vi "Auto Shooter Mode.vi"(0 "Shooter Command":T1, 7 "Current Angle":dbl, 9 "Ball Loaded?":bool) -> (8 "Secure Ball?":bool, 10 "Angle In Range?":bool, 11 "RPM Ready?":bool, 12 "Vision Target Aligned?":bool, 14 "State":T5, 15 "Shooter Ready?":bool, 16 "Left Output":dbl, 17 "Right Output":dbl, 18 "Angle Motor Output":dbl, 19 "Trigger Output":dbl)   [LabVIEW 2015]
uses:
  Common Code/Shooter State.ctl
  Common Code/Shooter Command Cluster.ctl
  Common Code/Shooter Commands.ctl
  Common Code/Shoot Modes Enum.ctl
  Common Code/Shot Type.ctl
  Common Code/Change Detect Int.vi
  Common Code/Change Detect Double.vi
  Robot Global Data.vi
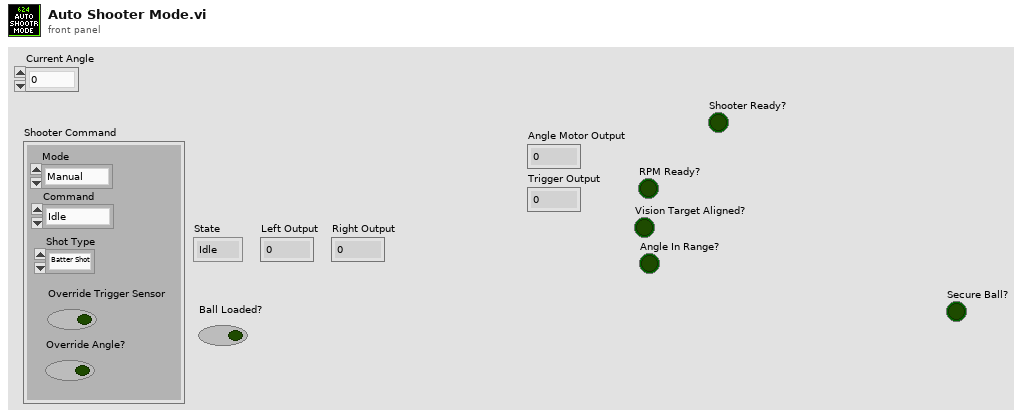
[diagram p1: front panel]
types:
  T1 = typedef "Shooter Command Cluster.ctl" = cluster{"Command":T2, "Mode":T3, "Shot Type":T4, "Override Trigger Sensor":bool, "Override Angle?":bool}
  T2 = typedef "Shooter Commands.ctl" = enum16{"Idle", "Prime Shooter", "Shoot"}
  T3 = typedef "Shoot Modes Enum.ctl" = enum16{"Manual", "Safe", "Auto"}
  T4 = typedef "Shot Type.ctl" = enum16{"Batter Shot", "Corner Shot", "Curve Shot", "Vision Shot", "Deep Middle Shot"}
  T5 = typedef "Shooter State.ctl" = enum16{"Idle", "Warmup", "Shooter Ready", "Shoot"}
  T6 = typedef "Dashboard Control Data.ctl" = cluster{"Shooter Presets":T7, "Encoder Control":T9, "Steer PID output":cluster{"output high":dbl, "output low":dbl}, " Steer PID gains":cluster{"proportional gain (Kc)":dbl, "integral time (Ti, min)":dbl, "derivative time (Td, min)":dbl}, "Drivetrain Settings":T10, "Vision Packet":T11, "Dashboard Drivetrain Command":T12, "Info/Command Cluster":T14, "Ball Vision Packet":T15, "Intake Presets":T17, "Intake Encoder Control":T19, "Climb Presets":T20, "Goal Output Range":cluster{"output high":dbl, "output low":dbl}, "Enabled Systems":T21, "Auton Presets":T22, "Pressure M":dbl, "Pressure B":dbl}
  T7 = typedef "Shooter Presets.ctl" = cluster{"Batter Shot":T8, "Deep Middle Shot":T8, "Manual Shot":T8, "Left Ticks Per Rotation":dbl, "Right Ticks Per Rotation":dbl, "Low Bar Shot":T8, "Shooter RPM Tolerance":dbl, "IIR Filter Power":dbl, "Trigger Power":dbl, "Fire from Load Delay":i32, "Max Angle":dbl, "Min Angle":dbl, "Angle PID gains":cluster{"P":dbl, "I":dbl, "D":dbl}, "Angle Output":cluster{"output high":dbl, "output low":dbl}, "Shooter Angle Tolerance":dbl, "Vision Shoot x^2":dbl, "Vision Shoot x":dbl, "Axis Camera Offset":dbl, "High Goal Center Height":dbl, "Feed Forward Max Accel":dbl, "Feed Forward Kv":dbl, "Backwards Trigger":dbl, "Shot Finish Delay (ms)":dbl, "Angle Max Current":dbl, "Angle Current Trip Time":dbl, "Intake Angle":dbl, "Vision Shoot c":dbl, "Reset?":bool, "Servo Release Delay":dbl, "Servo Idle Angle":i32, "Servo Hold Angle":i32, "Angle Pot x":dbl, "Angle Pot c":dbl, "Ignore Angle?":bool, "Manual Output?":bool, "Manual Out":dbl, "Max RPM":dbl, "Safty Frist Angle":dbl, "Intake Danger Height":dbl, "Angle Pot B":i32, "Angle Pot M":dbl, "FF Finish RPM":dbl, "RPM PID Right":cluster{"P":dbl, "I":dbl, "D":dbl, "FF":dbl}, "RPM PID Left":cluster{"P":dbl, "I":dbl, "D":dbl, "FF":dbl}, "Backwards RPM":dbl, "Vision RPM":dbl}
  T8 = typedef "Shot Presets.ctl" = cluster{"Left":dbl, "Right":dbl, "Angle":dbl}
  T9 = typedef "Encoder Control.ctl" = cluster{"Right Tick Constant":dbl, "Left Tick Constant":dbl, "Reset?":bool, "Y Dist":cluster{"PID gains":cluster{"proportional gain (Kc)":dbl, "integral time (Ti, min)":dbl, "derivative time (Td, min)":dbl}}, "Y Stop Thresh":dbl, "Y Stop Speed":dbl}
  T10 = typedef "Drivetrain Settings.ctl" = cluster{"Gyro Tolerance":dbl, "Throttle Ramp (ms)":dbl, "Angular rate compensation":bool, "Throttle to Rate Scale":dbl, "Rate compensation gain":dbl, "Kv":dbl, "Ka":dbl, "Feed Forward P":dbl, "Feed Forward D":dbl, "Goal Vision PID gains":cluster{"proportional gain (Kc)":dbl, "integral time (Ti, min)":dbl, "derivative time (Td, min)":dbl}, "Goal Detection Window":dbl, "Creep Rate":dbl}
  T11 = typedef "Goal Vision Packet.ctl" = cluster{"Distance":dbl, "Center X":dbl, "Center Y":dbl, "Found Target?":bool, "Robot Center":dbl, "Angle":dbl}
  T12 = typedef "Dashboard Drivetrain Command.ctl" = cluster{"Drivetrain Vision":T13}
  T13 = typedef "Drivetrain Vision.ctl" = cluster{"Goal Window":dbl, "Ball Window":dbl}
  T14 = typedef "Ball Tracking Command Cluster.ctl" = cluster{"Distance to Ball":dbl, "Desired Angle":dbl, "Command":enum16{"Turn to Ball", "Turn to Angle", "Get Distance"}, "Pixels from Center":dbl}
  T15 = typedef "Ball Vision Packet.ctl" = cluster{"Ball Detected?":bool, "Distance to Ball":dbl, "Desired Angle":dbl, "Pixels from Center":dbl, "Tracking mode":T16}
  T16 = typedef "Tracking Mode.ctl" = enum16{"Turn to Ball", "Turn to Angle"}
  T17 = typedef "Intake Presets.ctl" = cluster{"Intake Speed":dbl, "Outake Speed":dbl, "Low Height":dbl, "Half Height":dbl, "Full Height":dbl, "Angle Speed":dbl, "Angle Tolerance":dbl, "Encoder Scale":dbl, "Load Height":dbl, "Output Range":T18, "Rotation Power Max/Min":dbl, "MaxCurrent":dbl, "Intake Trip Time":dbl, "Idle Height":dbl, "Max Height":dbl, "Reset Encoders?":bool, "PID gains":cluster{"proportional gain (Kc)":dbl, "integral time (Ti, min)":dbl, "derivative time (Td, min)":dbl}}
  T18 = typedef "Drivetrain Output Range.ctl" = cluster{"output high":dbl, "output low":dbl}
  T19 = typedef "IntakeEcoderControl.ctl" = cluster{"Arm Tick Constant":dbl, "Reset?":bool, "Y Dist":cluster{"PID gains":cluster{"proportional gain (Kc)":dbl, "integral time (Ti, min)":dbl, "derivative time (Td, min)":dbl}}, "Y Stop Thresh":dbl, "Y Stop Speed":dbl}
  T20 = typedef "Climb Presets.ctl" = cluster{"Pull Power":dbl, "Time to Hold":dbl, "Extend Power":dbl}
  T21 = typedef "Enabled Systems.ctl" = cluster{"Shoot":bool, "Intake":bool, "DT":bool, "Gyro":bool, "100ms":bool, "US":bool}
  T22 = typedef "Autonomous Presets.ctl" = cluster{"Pitch Limit":dbl, "Roll Limit":dbl, "Ultrasonic Limit":dbl, "Start Position":dbl, "Cross Position":dbl}
  T23 = typedef "Intake Status Cluster.ctl" = cluster{"Roller Power":dbl, "Angle Power":dbl, "Intake Mode":T24, "Intake States":T25, "Rollers Active?":bool, "Current Height":dbl, "Target Height":dbl, "Encoder Raw Position":dbl, "Forward Tripped?":bool, "Backward Tripped?":bool, "Override IR?":bool}
  T24 = typedef "Intake Mode.ctl" = enum16{"Safe", "Auto", "Manual"}
  T25 = typedef "Intake States.ctl" = enum16{"Idle", "Set roller speed", "Move to angle"}
  T26 = typedef "Shooter State Cluster.ctl" = cluster{"State":T5, "Left RPM":dbl, "Right RPM":dbl, "Shooter Ready?":bool, "Ball Loaded?":bool, "Current Angle":dbl, "Angle Motor Output":dbl, "Trigger Output":dbl, "Angle Ready?":bool, "RPM Ready?":bool, "Vision Ready?":bool, "Ball Loaded?":bool, "Mode":T3, "Shot Type":T4, "Pot Height":dbl, "Current Tripped Forward?":bool, "Current Tripped Backward?":bool, "Right Servo":i32, "Left Servo":i32, "IR Override":bool, "Intake Danger?":bool}
  T27 = typedef "Drivetrain Status Cluster.ctl" = cluster{"Modes":T28, "Y (Throttle)":dbl, "X (Steer)":dbl, "Gyro In Range?":bool, "Distance Drive Finished?":bool, "Stop Eject Lockout":bool, "Dist Drive Status":T29, "Y Target":dbl, "Heading Target":dbl, "Vision Target Aligned?":bool, "Gear":dbl, "1st Gear Time":dbl, "2nd Gear Time":dbl, "1st Gear Shifts":dbl, "2nd Gear Shifts":dbl}
  T28 = typedef "Drivetrain Modes.ctl" = enum16{"Tank", "Climb", "Manual", "Goal Vision Targeting", "PID Distance Drive", "Hybrid", "Gyro Steer"}
  T29 = typedef "Dist Drive Status.ctl" = cluster{"Y In Range":bool, "X In Range":bool, "Gyro In Range":bool, "Y Dist":dbl, "X Dist":dbl, "Gyro":dbl}
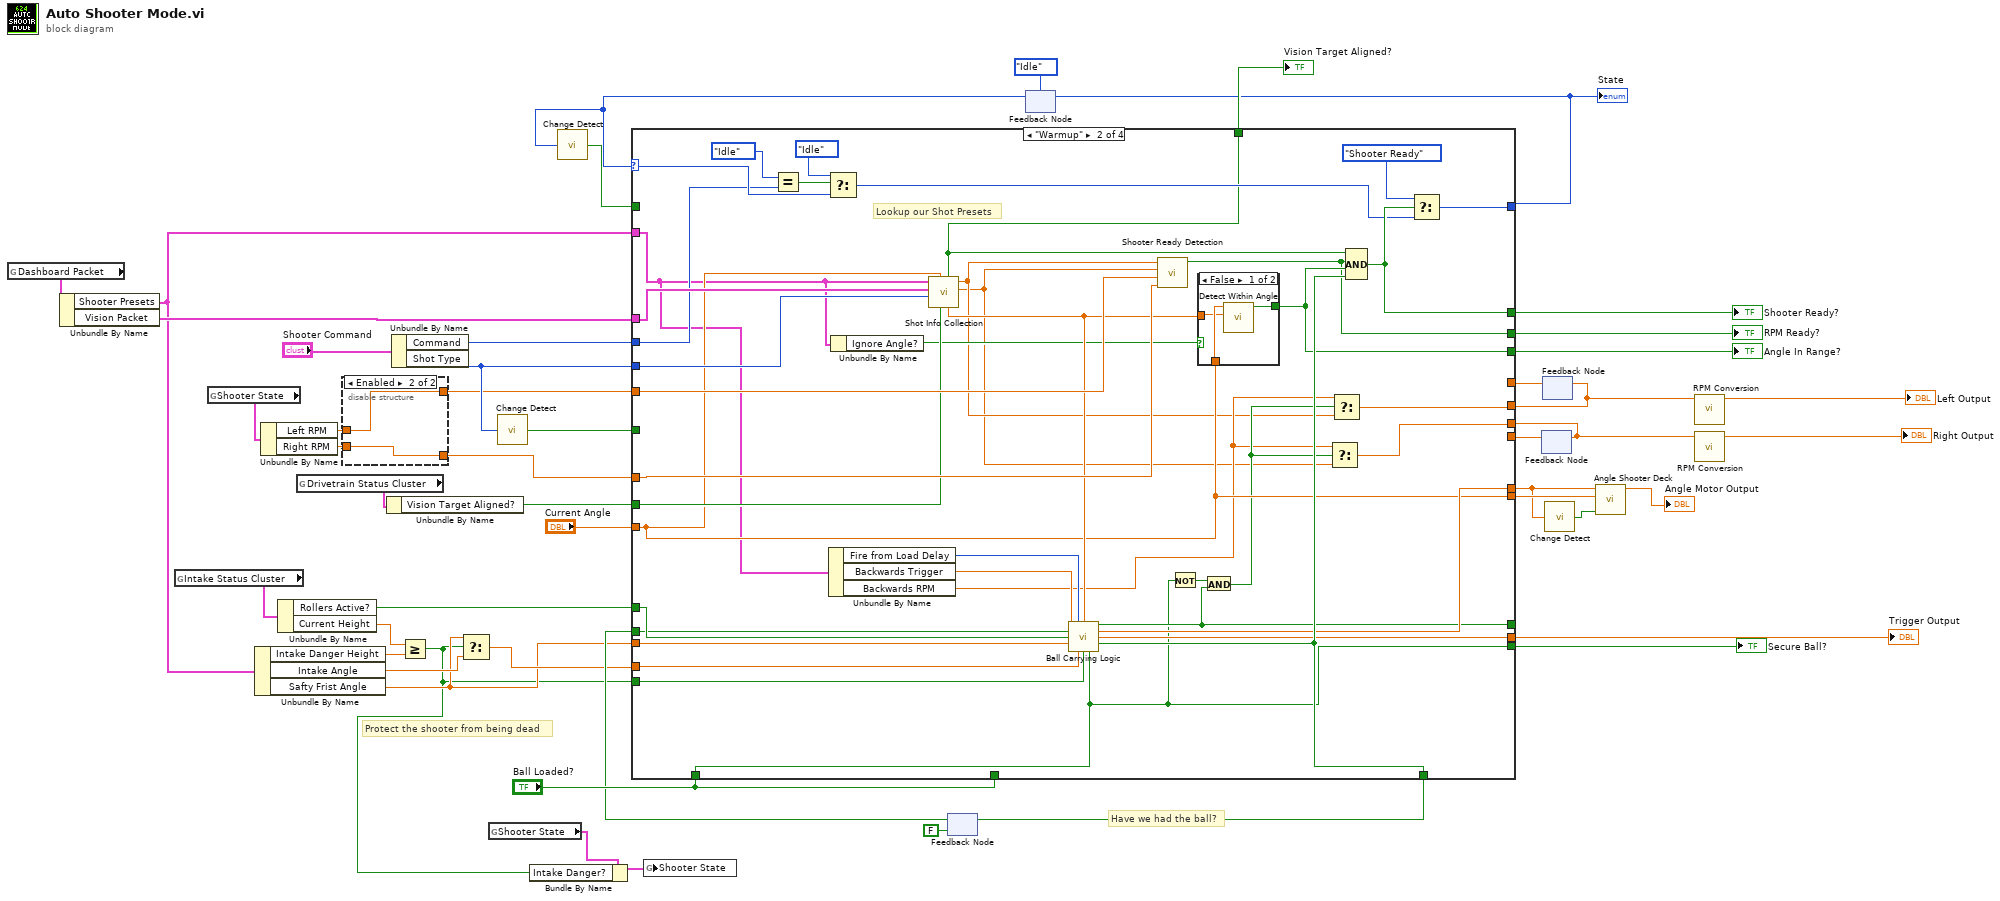
[diagram p0: block diagram]
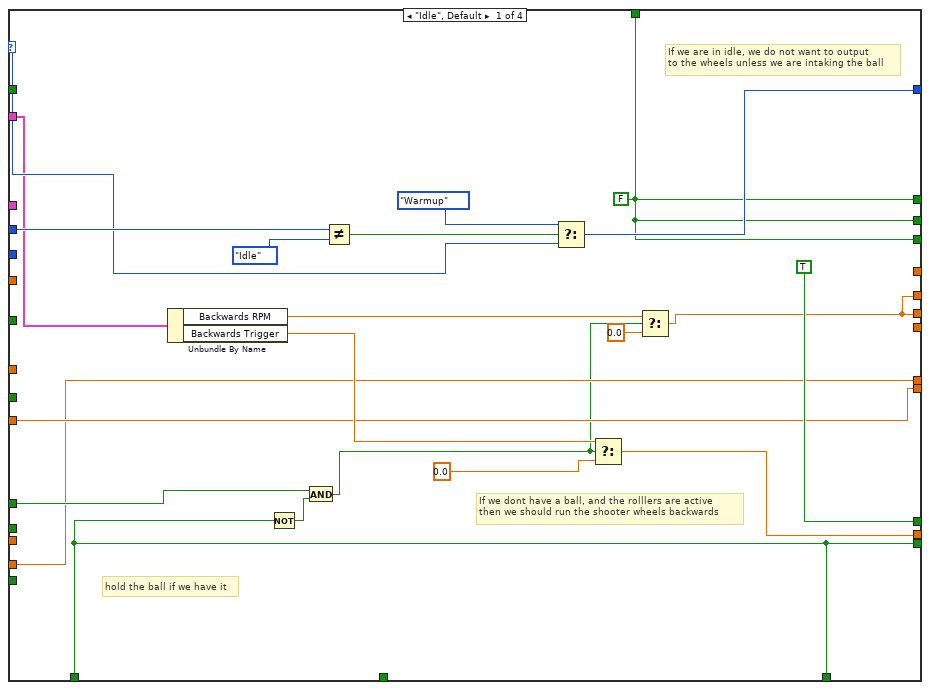
[diagram p3: hidden frame]
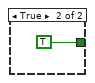
[diagram p4: hidden frame]
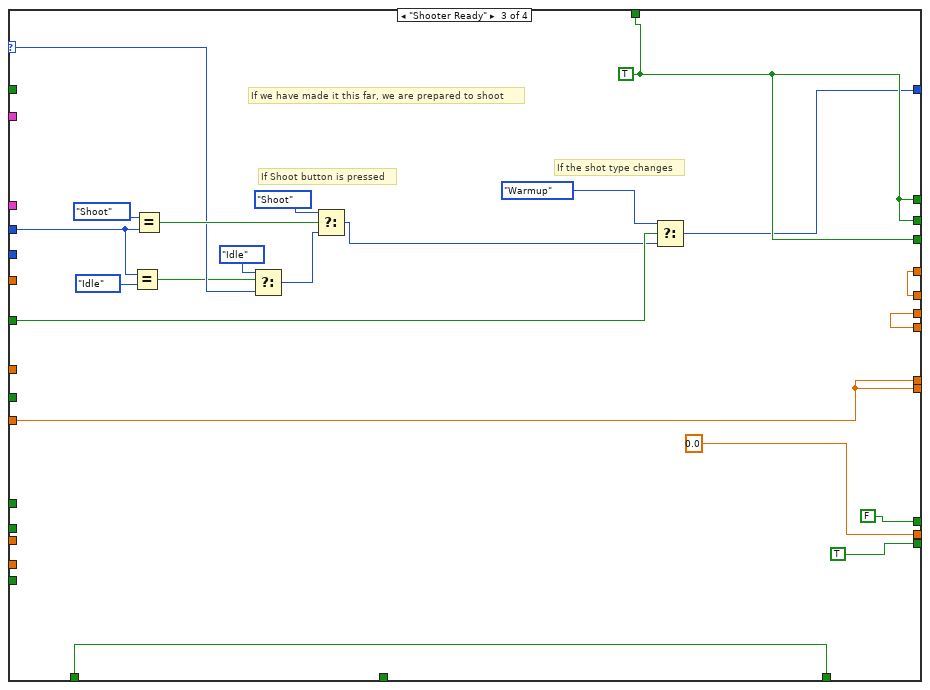
[diagram p5: hidden frame]
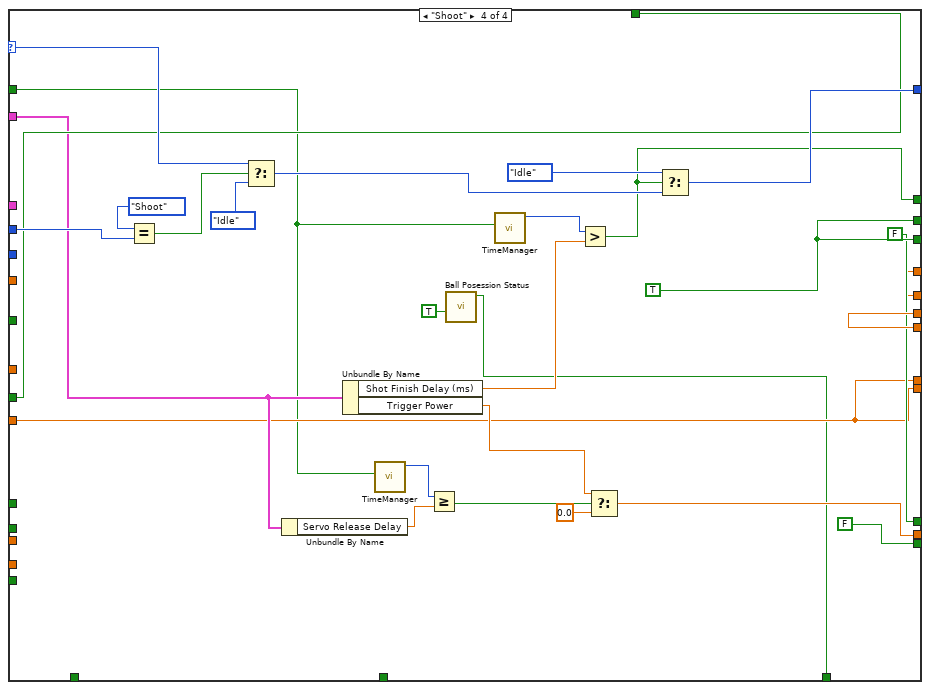
[diagram p6: hidden frame]
diagram:
  # "Protect the shooter from being dead"
  # "Have we had the ball?"
  n1 = global read "Robot Global Data.vi" "Dashboard Packet"() -> (w27:T6)
  n2 = Unbundle By Name(w27) -> ("Shooter Presets"=w26:T7, "Vision Packet"=w32:T11)
  n3 = global read "Robot Global Data.vi" "Intake Status Cluster"() -> (w25:T23)
  n4 = global read "Robot Global Data.vi" "Shooter State"() -> (w12:T26)
  n5 = Unbundle By Name(w26) -> ("Intake Danger Height"=w21:dbl, "Intake Angle"=w20:dbl, "Safty Frist Angle"=w18:dbl)
  n6 = Unbundle By Name(w12) -> ("Left RPM"=w11:dbl, "Right RPM"=w10:dbl)
  n7 = Unbundle By Name(w25) -> ("Rollers Active?"=w40:bool, "Current Height"=w22:dbl)
  n8 = global read "Robot Global Data.vi" "Drivetrain Status Cluster"() -> (w42:T27)
  n9 = disable-structure shown="Enabled" {
    disable-tunnel: [w50 w52] -> w17
    disable-tunnel: [_ w51] -> w16
    disable-tunnel: w11 -> [_ w52]
    disable-tunnel: w10 -> [_ w51]
    frame Disabled {
    }
    frame Enabled {
    }
  }
  n10 = Unbundle By Name(w42) -> ("Vision Target Aligned?"=w41:bool)
  n11 = Unbundle By Name("Shooter Command") -> ("Command"=w48:T2, "Shot Type"=w46:T4)
  n12 = Greater Or Equal?(x=w22, y=w21) -> (x >= y?=w1:bool)
  n13 = Select(t=w18, s=w1, f=w20) -> (s? t:f=w19:dbl)
  n14 = global read "Robot Global Data.vi" "Shooter State"() -> (w3:T26)
  n15 = call-poly "Change Detect.vi"("In"=w46) -> ("Changed?"=w45:bool)
  n16 = Bundle By Name(cluster=w3, "Intake Danger?"=w1) -> (w2:T26)
  n17 = global write "Robot Global Data.vi" "Shooter State"(w2) -> ()
  n18 = feedback #1(FALSE ("Ball Loaded?")) -> (w37:bool)
  n19 = feedback #2(Shooter_State."Idle") -> (w35:T5)
  n20 = call-poly "Change Detect.vi"("In"=w35) -> ("Changed?"=w34:bool)
  n21 = feedback #3() -> (w43:dbl)  [unwired: 1 in]
  n22 = feedback #4() -> (w44:dbl)  [unwired: 1 in]
  n23 = case shown="\"Warmup\"" w35 {
    selector: w35 -> [w68 w101 w127 w163]
    tunnel: w48 -> [w69 w98 w134 w166]
    tunnel: [w71 w111 w119 w159] -> w23
    tunnel: w26 -> [w58 w84 _ w151]
    tunnel: w46 -> [_ w113 _ _]
    tunnel: [w53 w77 w135 w162] -> w7
    tunnel: [w53 w76 w118 w142] -> w9
    tunnel: w45 -> [_ _ w137 _]
    tunnel: w44 -> [_ _ w118 w142]
    tunnel: w43 -> [_ _ w135 w162]
    tunnel: w17 -> [_ w110 _ _]
    tunnel: w16 -> [_ w109 _ _]
    tunnel: w41 -> [_ w106 _ w156]
    tunnel: "Ball Loaded?" -> [_ _ _ _]
    tunnel: w32 -> [_ w108 _ _]
    tunnel: [w60 w91 w120 w143] -> w5
    tunnel: w40 -> [w66 w104 _ _]
    tunnel: [w63 w93 0.0 ("f") w145] -> w13
    tunnel: "Ball Loaded?" -> [w57 w75 w133 _]
    tunnel: [w57 w105 w133 w140] -> w38
    tunnel: w37 -> [_ w74 _ _]
    tunnel: w34 -> [_ _ _ w141]
    tunnel: "Current Angle" -> [w61 w86 w120 w143]
    tunnel: [w59 w107 w123 w152] -> w31
    tunnel: [w59 w95 w123 w157] -> w30
    tunnel: [w59 w94 w123 w157] -> w29
    tunnel: [w59 w85 w123 w156] -> w28
    tunnel: [TRUE w82 FALSE FALSE] -> _
    tunnel: w19 -> [w60 w90 _ _]
    tunnel: [w57 w75 TRUE ("Intake High Angle Allowed?") FALSE ("Intake High Angle Allowed?")] -> w24
    tunnel: w1 -> [_ w88 _ _]
    tunnel: w18 -> [_ w87 _ _]
    tunnel: [w61 w86 w120 w143] -> w14
    frame "Idle", Default {
      w59 = FALSE ("Shooter Ready?")
      # "hold the ball if we have it"
      # "If we dont have a ball, and the rolllers are active\nthen we should run the shooter wheels backwards"
      # "If we are in idle, we do not want to output\nto the wheels unless we are intaking the ball"
      n24 = Unbundle By Name(w58) -> ("Backwards RPM"=w54:dbl, "Backwards Trigger"=w64:dbl)
      n25 = Not(x=w57) -> (.not. x?=w65:bool)
      n26 = And(x=w66, y=w65) -> (x .and. y?=w56:bool)
      n27 = Not Equal?(x=w69, y=Shooter_Commands."Idle" ("Command")) -> (x != y?=w72:bool)
      n28 = Select(t=Shooter_State."Warmup", s=w72, f=w68) -> (s? t:f=w71:T5)
      n29 = Select(t=w64, s=w56, f=0.0) -> (s? t:f=w63:dbl)
      n30 = Select(t=w54, s=w56, f=0.0) -> (s? t:f=w53:dbl)
    }
    frame "Warmup" {
      # "Lookup our Shot Presets"
      n31 = Equal?(x=Shooter_Commands."Idle" ("y"), y=w98) -> (x = y?=w99:bool)
      n32 = Select(t=Shooter_State."Idle", s=w99, f=w101) -> (s? t:f=w100:T5)
      n33 = Unbundle By Name(w84) -> ("Fire from Load Delay"=w103:i32, "Backwards Trigger"=w102:dbl, "Backwards RPM"=w80:dbl)
      n34 = Unbundle By Name(w84) -> ("Ignore Angle?"=w89:bool)
      n35 = call "Shot Info Collection.vi"("Vision Target Aligned? in"=w106, "Current Angle"=w86, "Shot Type"=w113, "Vision Packet"=w108, "Shooter Presets"=w84) -> ("Right Wheel RPM"=w78:dbl, "Left Wheel RPM"=w79:dbl, "Angle"=w92:dbl, "Vision Target Aligned? out"=w85:bool)  [unwired: 3 in]
      n36 = call "Ball Carrying Logic.vi"("Backwards Trigger"=w102, "Fire from Load Delay"=w103, "Angle in"=w92, "Had Ball Before?"=w74, "Rollers Active? in"=w104, "Safty Frist Angle"=w87, "Intake Angle"=w90, "Intake at Dangerous Height?"=w88, "Ball Loaded? in"=w75) -> ("Rollers Active? out"=w82:bool, "Angle out"=w91:dbl, "Trigger Out"=w93:dbl, "Ball Loaded? out"=w105:bool)  [unwired: 3 in]
      n37 = call "Shooter Ready Detection.vi"("Right RPM"=w109, "Left RPM"=w110, "Right RPM Target"=w78, "Left RPM Target"=w79) -> ("Shooter Ready?"=w94:bool)  [unwired: 7 in]
      n38 = Not(x=w75) -> (.not. x?=w83:bool)
      n39 = case shown="False" w89 {
        tunnel: [w116 TRUE ("In Range?")] -> w95
        tunnel: w86 -> [w115 _]
        tunnel: w92 -> [w114 _]
        frame False {
          n40 = call "Detect Within Angle.vi"("Angle Target"=w114, "Current Angle"=w115) -> ("In Range?"=w116:bool)  [unwired: 9 in]
        }
        frame True {
        }
      }
      n41 = And(x=w83, y=w82) -> (x .and. y?=w81:bool)
      n42 = Select(t=w80, s=w81, f=w78) -> (s? t:f=w77:dbl)
      n43 = Select(t=w80, s=w81, f=w79) -> (s? t:f=w76:dbl)
      n44 = Compound Arithmetic op=AND(w85, w94, w95, w105) -> (w107:bool)
      n45 = Select(t=Shooter_State."Shooter Ready", s=w107, f=w100) -> (s? t:f=w111:T5)
    }
    frame "Shooter Ready" {
      w123 = TRUE ("Vision Target Aligned?")
      # "If the shot type changes"
      # "If Shoot button is pressed"
      # "If we have made it this far, we are prepared to shoot"
      n46 = Equal?(x=w134, y=Shooter_Commands."Idle") -> (x = y?=w126:bool)
      n47 = Equal?(x=Shooter_Commands."Shoot", y=w134) -> (x = y?=w132:bool)
      n48 = Select(t=Shooter_State."Idle", s=w126, f=w127) -> (s? t:f=w128:T5)
      n49 = Select(t=Shooter_State."Shoot", s=w132, f=w128) -> (s? t:f=w130:T5)
      n50 = Select(t=Shooter_State."Warmup", s=w137, f=w130) -> (s? t:f=w119:T5)
    }
    frame "Shoot" {
      w157 = TRUE ("Vision Target Aligned?")
      n51 = Equal?(x=Shooter_Commands."Shoot", y=w166) -> (x = y?=w164:bool)
      n52 = Select(t=w163, s=w164, f=Shooter_State."Idle") -> (s? t:f=w160:T5)
      n53 = Unbundle By Name(w151) -> ("Servo Release Delay"=w150:dbl)
      n54 = Unbundle By Name(w151) -> ("Shot Finish Delay (ms)"=w154:dbl, "Trigger Power"=w147:dbl)
      n55 = call "TimeManager.vi"("Reset?"=w141) -> ("Time Since Reset"=w149:u32)  [unwired: 9 in, 1 out]
      n56 = Greater Or Equal?(x=w149, y=w150) -> (x >= y?=w148:bool)
      n57 = call "Ball Posession Status.vi"("Logical Exit?"=TRUE) -> ("Ball Posessed?"=w140:bool)  [unwired: 10 in]
      n58 = call "TimeManager.vi"("Reset?"=w141) -> ("Time Since Reset"=w153:u32)  [unwired: 9 in, 1 out]
      n59 = Greater?(x=w153, y=w154) -> (0:w152:bool)
      n60 = Select(t=w147, s=w148, f=0.0) -> (s? t:f=w145:dbl)
      n61 = Select(t=Shooter_State."Idle" ("f"), s=w152, f=w160) -> (s? t:f=w159:T5)
    }
  }
  "State" <- w23
  "Trigger Output" <- w13
  "Shooter Ready?" <- w31
  "RPM Ready?" <- w29
  "Angle In Range?" <- w30
  "Vision Target Aligned?" <- w28
  "Secure Ball?" <- w24
  n62 = feedback-in #1(w38) -> ()
  n63 = feedback-in #2(w23) -> ()
  n64 = feedback-in #3(w7) -> ()
  n65 = feedback-in #4(w9) -> ()
  n66 = call-poly "Change Detect.vi"("In"=w5) -> ("Changed?"=w4:bool)
  n67 = call "Angle Shooter Deck.vi"("reinitialize? (F)"=w4, "Shooter Angle"=w14, "Target Angle"=w5) -> ("Angle Motor Power Out"=→"Angle Motor Output":dbl)  [unwired: 8 in]
  n68 = call "RPM Conversion.vi"("RPM"=w9) -> ("RPM Out"=→"Left Output":dbl)  [unwired: 10 in]
  n69 = call "RPM Conversion.vi"("RPM"=w7) -> ("RPM Out"=→"Right Output":dbl)  [unwired: 10 in]
